vi "PreLoop.vi"(11 "Actor":refnum<class "Actor.lvclass">) -> (2 "EventRegRef":refnum<event-registration>, 3 "Actor":refnum<class "Actor.lvclass">)   [LabVIEW 2020, in "jettl.lvlib"]
uses:
  jettl.lvlib
  Actor/Actor.lvclass
  Msg/Msg.lvclass
  Msg.ctl
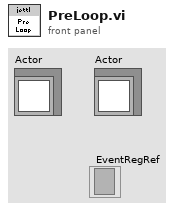
[diagram p1: front panel]
types:
  T1 = typedef "jettl.lvlib/Base.ctl" = cluster{"State":T2, "SelfUnified":T4, "ParentUnified":T4, "ChildUnifiedMap":T6}
  T2 = typedef "jettl.lvlib/State.ctl" = cluster{"Lifecycle":T3}
  T3 = typedef "jettl.lvlib/Lifecycle.ctl" = enum16{"Initializing", "SettingUp", "Starting", "Running", "Stopping", "TearingDown", "Terminated"}
  T4 = typedef "jettl.lvlib/Unified.ctl" = cluster{"Alias":string, "MsgSet":T5, "Root":bool, "Leaf":bool, "MsgDVREvent":refnum<user-event>, "EventRegRef":refnum<event-registration>, "PreSetupQueue":refnum<queue>, "BeginSetupQueue":refnum<queue>, "PostSetupQueue":refnum<queue>, "VIRef":refnum<vi>, "DestroyQueue":refnum<queue>}
  T5 = typedef "jettl.lvlib/MsgSet.ctl" = set{refnum<class "Msg.lvclass">}
  T6 = typedef "jettl.lvlib/ChildUnifiedMap.ctl" = map{string, T4}
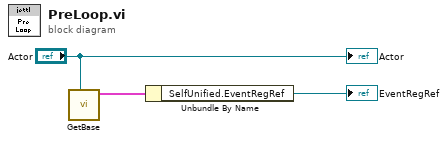
[diagram p0: block diagram]
diagram:
  n1 = call-dynamic "GetBase.vi"("Actor"="Actor") -> ("BaseActor"=w3:T1)  [unwired: 10 in]
  n2 = Unbundle By Name(w3) -> ("SelfUnified.EventRegRef"=→"EventRegRef":refnum<event-registration>)
  "Actor" <- "Actor"
